vi "gentec-M-Link.Query Sensor Type.vi"(0 "VISA resource In":refnum<visa-resource-name>, 5 "error in (no error)":errorcluster) -> (11 "Data Read":string, 13 "Read Timeout":bool, 14 "VISA resource Out":refnum<visa-resource-name>, 16 "Sensor Type":T1=1 items=["unknown", "Radiometer", "Joule Meter", "Optical Power", "Thermopyle Power"], 19 "error out":errorcluster)   [LabVIEW 2014, in "gentec-M-Link - Driver.lvlib"]
doc: "Data to write: pty"
uses:
  gentec-M-Link - Driver.lvlib
  Type Defs/gentec-M-Link.Sensor Type.ctl
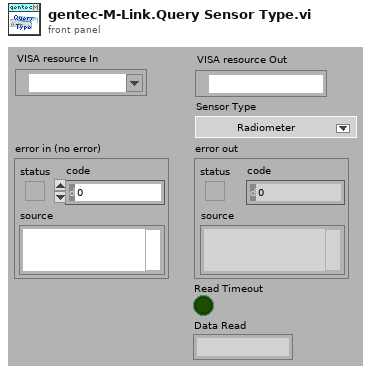
[diagram p1: front panel]
types:
  T1 = typedef "gentec-M-Link - Driver.lvlib/gentec-M-Link.Sensor Type.ctl" = u16
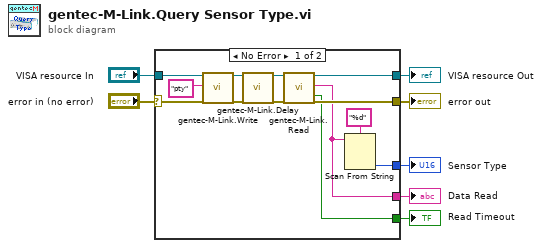
[diagram p0: block diagram]
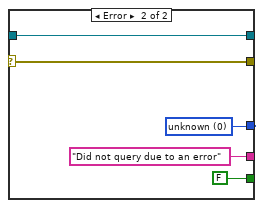
[diagram p2: hidden frame]
diagram:
  n1 = case shown="No Error" "error in (no error)" {
    selector: "error in (no error)" -> [w15 w25]
    tunnel: [w19 w25] -> w6
    tunnel: "VISA resource In" -> [w16 w24]
    tunnel: [w17 w24] -> w4
    tunnel: [w13 "Did not query due to an error" ("Data Read")] -> w3
    tunnel: [w12 FALSE ("Read Timeout")] -> w2
    tunnel: [w11 w21] -> w1
    frame No Error {
      n2 = call "gentec-M-Link.Write.vi"("VISA resource (In)"=w16, "Data To Write"="pty", "error in (no error)"=w15) -> ("VISA resource (Out)"=w9:refnum<visa-resource-name>, "error out"=w14:errorcluster)  [unwired: 14 in, 1 out]
      n3 = call "gentec-M-Link.Delay.vi"("VISA resource In"=w9, "error in (no error)"=w14) -> ("VISA resource Out"=w8:refnum<visa-resource-name>, "error out"=w10:errorcluster)  [unwired: 16 in]
      n4 = call "gentec-M-Link.Read.vi"("VISA resource (In)"=w8, "error in (no error)"=w10) -> ("VISA resource (Out)"=w17:refnum<visa-resource-name>, "Data Read"=w13:string, "Read Timeout"=w12:bool, "error out"=w19:errorcluster)  [unwired: 13 in, 1 out]
      n5 = Scan From String(format string="%d", input string=w13) -> (output 1=w11:i32)  [unwired: 3 in, 3 out]
    }
    frame Error {
      w21 = T1 0 items=["unknown", "Radiometer", "Joule Meter", "Optical Power", "Thermopyle Power"] ("Sensor Type")
    }
  }
  "error out" <- w6
  "VISA resource Out" <- w4
  "Sensor Type" <- w1
  "Data Read" <- w3
  "Read Timeout" <- w2
